vi "VariousControlsForLift.vi"(10 "State":T2(ring)) -> (1 "Lift Motor Right":dbl=0.5, 2 "Lift Motor Left":dbl=-0.25, 3 "State Out":T2(ring)=enum."Three Tote")   [LabVIEW 2014]
uses:
  Global Variables.vi
  <vilib>/addons/control/pid/pid.llb/PID (DBL).vi
  <vilib>/addons/control/pid/NI_PID_pid.lvlib
panel:
  in  "PID right":T1={"proportional gain (Kc)"=1.0, "integral time (Ti, min)"=0.01, "derivative time (Td, min)"=0.0} {"derivative time (Td, min)" format="%.3f"; "integral time (Ti, min)" format="%.10f"; "proportional gain (Kc)" format="%.3f"}
  in  "right slave output range":cluster{"output high":dbl, "output low":dbl}={"output high"=0.5, "output low"=-0.5} {"output low" format="%.2f"; "output high" format="%.2f"}
  in  "left master output range":cluster{"output high":dbl, "output low":dbl}={"output high"=0.25, "output low"=-0.25} {"output low" format="%.2f"; "output high" format="%.2f"}
  out "Encoder":dbl=310.75
  in  "PID left":T1={"proportional gain (Kc)"=0.006, "integral time (Ti, min)"=0.0, "derivative time (Td, min)"=0.0} {"derivative time (Td, min)" format="%.3f"; "integral time (Ti, min)" format="%.3f"; "proportional gain (Kc)" format="%.3f"}
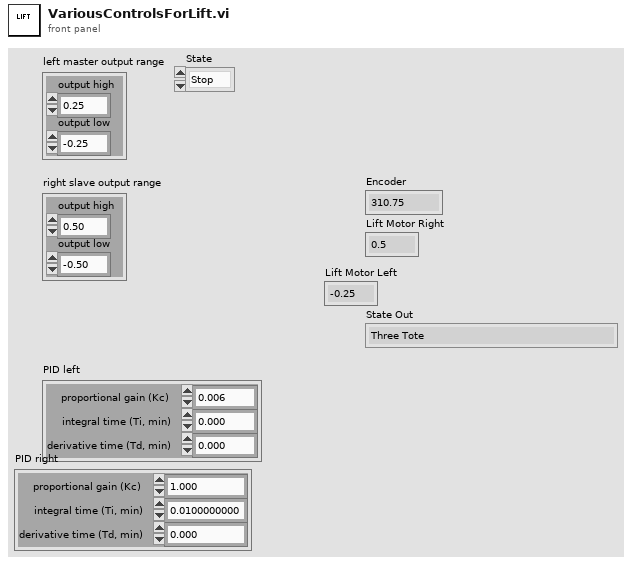
[diagram p1: front panel]
types:
  T1 = cluster{"proportional gain (Kc)":dbl, "integral time (Ti, min)":dbl, "derivative time (Td, min)":dbl}
  T2 = enum16{"Stop", "Three Tote", "Two Tote", "One Tote", "Step", "Top", "Home", "Joystick", "Joystick Slave", "D Pad"}
  T3 = typedef "WPI_EncoderDevRef.ctl" = cluster{"DevStatus":errorcluster, "EncoderIndex":T4, "CounterIndex":T5, "DistancePerCount":dbl, "Decoding Type":T6}
  T4 = typedef "FPGA_EncoderIdx.ctl" = enum8{"Enc 0", "Enc 1", "Enc 2", "Enc 3", "Enc 4", "Enc 5", "Enc 6", "Enc 7", "Invalid"}
  T5 = typedef "FPGA_CounterCtrSystemIndex.ctl" = enum8{"Ctr 0", "Ctr 1", "Ctr 2", "Ctr 3", "Ctr 4", "Ctr 5", "Ctr 6", "Ctr 7", "Invalid"}
  T6 = typedef "WPI_EncoderType.ctl" = enum16{"1x", "2x", "4x"}
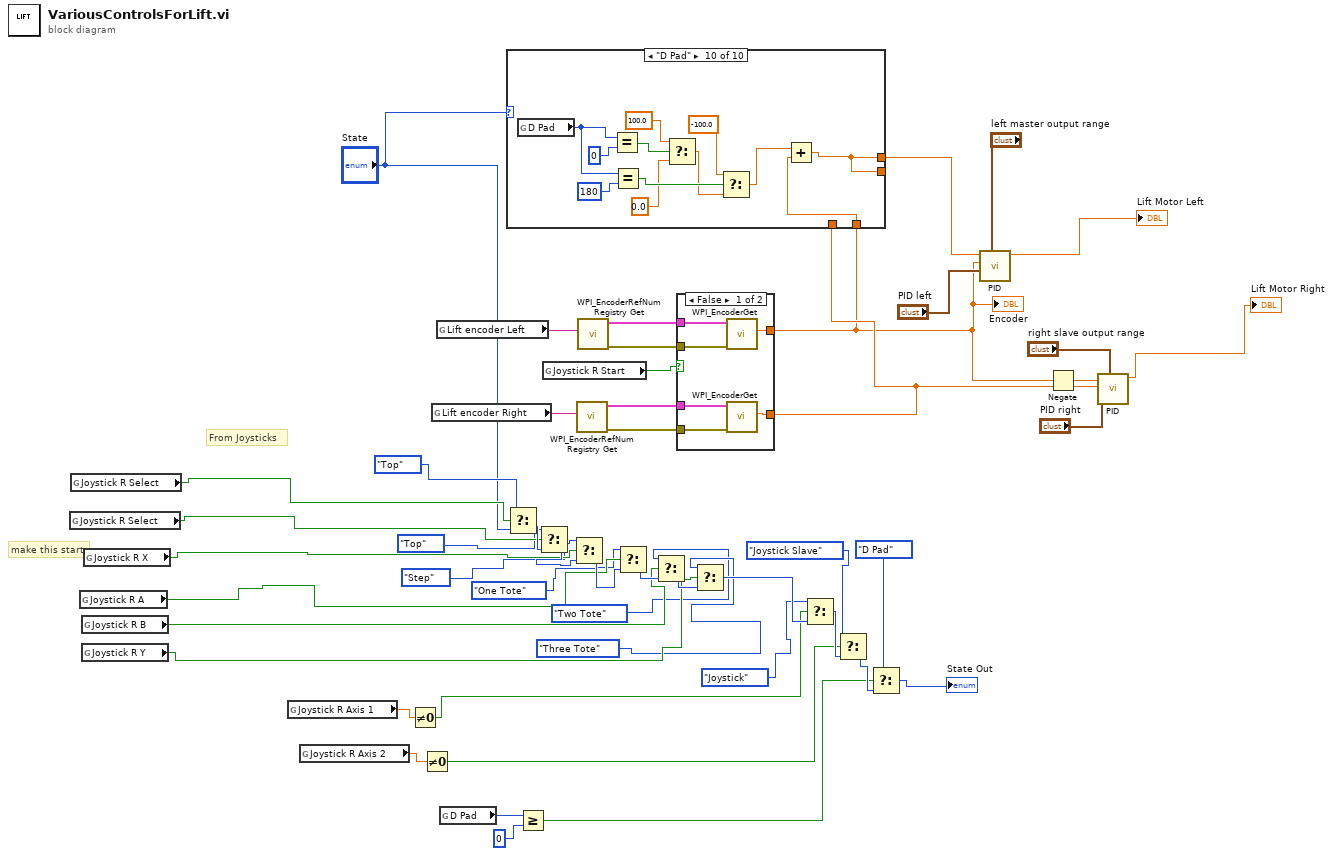
[diagram p0: block diagram]
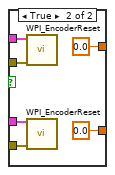
[diagram p2: hidden frame]
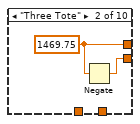
[diagram p4: hidden frame]
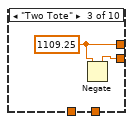
[diagram p5: hidden frame]
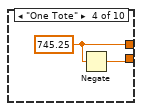
[diagram p6: hidden frame]
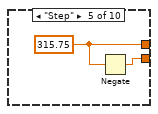
[diagram p7: hidden frame]
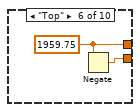
[diagram p8: hidden frame]
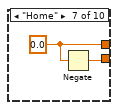
[diagram p9: hidden frame]
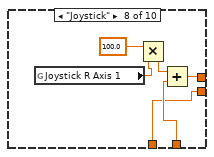
[diagram p10: hidden frame]
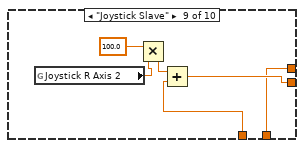
[diagram p11: hidden frame]
diagram:
  # "make this start"
  # "From Joysticks"
  n1 = global read "Global Variables.vi" "Joystick R Select"() -> (w35:bool)
  n2 = global read "Global Variables.vi" "Joystick R Select"() -> (w36:bool)
  n3 = global read "Global Variables.vi" "Joystick R A"() -> (w40:bool)
  n4 = global read "Global Variables.vi" "Joystick R B"() -> (w39:bool)
  n5 = global read "Global Variables.vi" "Joystick R Y"() -> (w38:bool)
  n6 = global read "Global Variables.vi" "Joystick R X"() -> (w37:bool)
  n7 = global read "Global Variables.vi" "Joystick R Axis 1"() -> (w33:dbl)
  n8 = global read "Global Variables.vi" "Joystick R Axis 2"() -> (w19:dbl)
  n9 = Not Equal To 0?(x=w33) -> (x != 0?=w34:bool)
  n10 = Not Equal To 0?(x=w19) -> (x != 0?=w27:bool)
  n11 = global read "Global Variables.vi" "Lift encoder Right"() -> (w32:string)
  n12 = global read "Global Variables.vi" "Lift encoder Left"() -> (w42:string)
  n13 = global read "Global Variables.vi" "D Pad"() -> (w11:i16)
  n14 = Select(t=T2."Top" ("State Out"), s=w36, f="State") -> (s? t:f=w49:T2)
  n15 = Greater Or Equal?(x=w11, y=i16 0) -> (x >= y?=w8:bool)
  n16 = Select(t=T2."Top" ("State Out"), s=w35, f=w49) -> (s? t:f=w48:T2)
  n17 = global read "Global Variables.vi" "Joystick R Start"() -> (w2:bool)
  n18 = Select(t=T2."Step" ("State Out"), s=w37, f=w48) -> (s? t:f=w47:T2)
  n19 = call <vilib>:"WPI_EncoderRefNum Registry Get.vi"("refnum name"=w32) -> ("error out"=w30:errorcluster, "EncoderDevRef"=w31:T3)  [unwired: 9 in]
  n20 = call <vilib>:"WPI_EncoderRefNum Registry Get.vi"("refnum name"=w42) -> ("error out"=w44:errorcluster, "EncoderDevRef"=w43:T3)  [unwired: 9 in]
  n21 = Select(t=T2."One Tote" ("State Out"), s=w40, f=w47) -> (s? t:f=w46:T2)
  n22 = Select(t=T2."Two Tote" ("State Out"), s=w39, f=w46) -> (s? t:f=w45:T2)
  n23 = case shown="False" w2 {
    tunnel: w44 -> [w55 w60]
    tunnel: w43 -> [w54 w59]
    tunnel: w31 -> [w53 w58]
    tunnel: w30 -> [w52 w61]
    tunnel: [w51 0.0 ("Distance")] -> w1
    tunnel: [w50 0.0 ("Distance")] -> w16
    frame False {
      n24 = call <vilib>:"WPI_EncoderGet.vi"("error in (no error)"=w55, "EncoderDevRef"=w54) -> ("Distance"=w51:dbl)  [unwired: 4 in, 5 out]
      n25 = call <vilib>:"WPI_EncoderGet.vi"("error in (no error)"=w52, "EncoderDevRef"=w53) -> ("Distance"=w50:dbl)  [unwired: 4 in, 5 out]
    }
    frame True {
      n26 = call <vilib>:"WPI_EncoderReset.vi"("error in (no error)"=w60, "EncoderDevRef"=w59) -> ()  [unwired: 8 in, 2 out]
      n27 = call <vilib>:"WPI_EncoderReset.vi"("error in (no error)"=w61, "EncoderDevRef"=w58) -> ()  [unwired: 8 in, 2 out]
    }
  }
  "Encoder" <- w1
  n28 = case shown="\"D Pad\"" "State" {
    tunnel: [w63 w64 w67 w68 w70 w72 w74 w81 w82 w88] -> w18
    tunnel: w1 -> [w63 _ _ _ _ _ _ w80 w82 w89]
    tunnel: w16 -> [w62 _ _ _ _ _ _ w76 w84 _]
    tunnel: [w62 w65 w66 w69 w71 w73 w75 w76 w83 w88] -> _
    frame "Stop", Default {
    }
    frame "Three Tote" {
      w64 = 1469.75 ("setpoint")
      n29 = Negate(x=w64) -> (-x=w65:dbl)
    }
    frame "Two Tote" {
      w67 = 1109.25 ("setpoint")
      n30 = Negate(x=w67) -> (-x=w66:dbl)
    }
    frame "One Tote" {
      w68 = 745.25 ("setpoint")
      n31 = Negate(x=w68) -> (-x=w69:dbl)
    }
    frame "Step" {
      w70 = 315.75 ("setpoint")
      n32 = Negate(x=w70) -> (-x=w71:dbl)
    }
    frame "Top" {
      w72 = 1959.75 ("setpoint")
      n33 = Negate(x=w72) -> (-x=w73:dbl)
    }
    frame "Home" {
      w74 = 0.0 ("setpoint")
      n34 = Negate(x=w74) -> (-x=w75:dbl)
    }
    frame "Joystick" {
      n35 = global read "Global Variables.vi" "Joystick R Axis 1"() -> (w77:dbl)
      n36 = Multiply(x=100.0, y=w77) -> (x*y=w79:dbl)
      n37 = Add(x=w79, y=w80) -> (x+y=w81:dbl)
    }
    frame "Joystick Slave" {
      n38 = global read "Global Variables.vi" "Joystick R Axis 2"() -> (w85:dbl)
      n39 = Multiply(x=100.0, y=w85) -> (x*y=w87:dbl)
      n40 = Add(x=w87, y=w84) -> (x+y=w83:dbl)
    }
    frame "D Pad" {
      n41 = global read "Global Variables.vi" "D Pad"() -> (w97:i16)
      n42 = Equal?(x=w97, y=i16 0) -> (x = y?=w96:bool)
      n43 = Equal?(x=w97, y=i16 180) -> (x = y?=w95:bool)
      n44 = Select(t=100.0, s=w96, f=0.0) -> (s? t:f=w94:dbl)
      n45 = Select(t=-100.0, s=w95, f=w94) -> (s? t:f=w91:dbl)
      n46 = Add(x=w91, y=w89) -> (x+y=w88:dbl)
    }
  }
  n47 = Select(t=T2."Three Tote" ("State Out"), s=w38, f=w45) -> (s? t:f=w41:T2)
  n48 = Select(t=T2."Joystick" ("State Out"), s=w34, f=w41) -> (s? t:f=w28:T2)
  n49 = Select(t=T2."Joystick Slave" ("State Out"), s=w27, f=w28) -> (s? t:f=w9:T2)
  n50 = Select(t=T2."D Pad", s=w8, f=w9) -> (s? t:f=→"State Out":T2)
  n51 = call-poly <vilib>:"PID.vi"("output range"="left master output range", "PID gains"="PID left", "process variable"=w1, "setpoint"=w18) -> ("output"=→"Lift Motor Left":dbl)  [unwired: 6 in, 1 out]
  n52 = Negate(x=w1) -> (-x=w4:dbl)
  n53 = call-poly <vilib>:"PID.vi"("output range"="right slave output range", "PID gains"="PID right", "process variable"=w16, "setpoint"=w4) -> ("output"=→"Lift Motor Right":dbl)  [unwired: 6 in, 1 out]
